vi "Execute.vi"(8 "error in (no error)":errorcluster, 11 "Node in":refnum<class "bt_Selector.lvclass">) -> (0 "error out":errorcluster, 1 "Status":T1, 3 "Node out":refnum<class "bt_Selector.lvclass">)   [LabVIEW 2021, in "BT.lvlib" / "bt_Selector.lvclass"]
uses:
  bt_Selector.lvclass
  bt_Selector.lvclass/bt_Selector.ctl
  abs_Node/Status.ctl
  abs_Node/bt_Node.lvclass
  abs_Composite/bt_Composite.lvclass
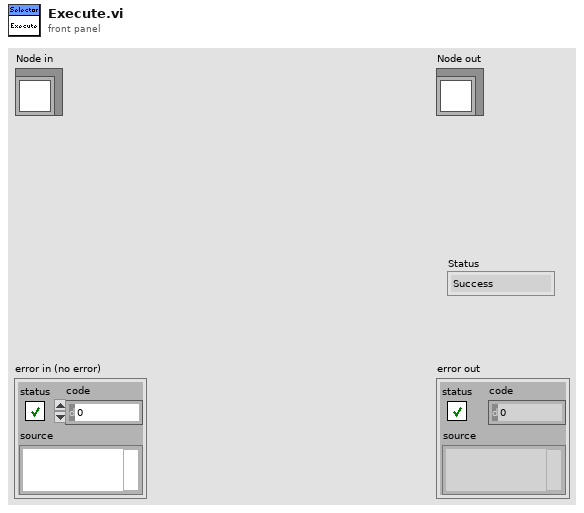
[diagram p1: front panel]
types:
  T1 = typedef "BT.lvlib/bt_Node.lvclass/Status.ctl" = enum16{"Success", "Failure", "Running"}
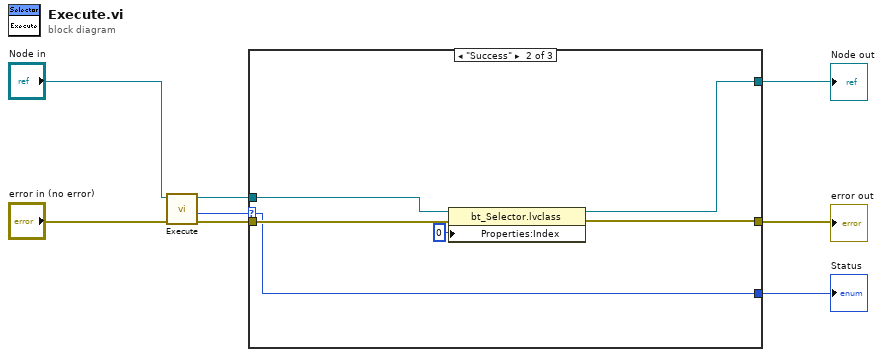
[diagram p0: block diagram]
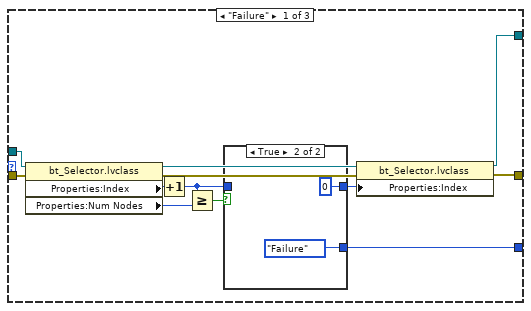
[diagram p2: hidden frame]
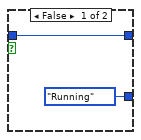
[diagram p3: hidden frame]
diagram:
  n1 = call-parent "Execute.vi"("error in (no error)"="error in (no error)", "Node in"="Node in") -> ("error out"=w3:errorcluster, "Status"=w1:T1, "Node out"=w2:refnum<class "bt_Selector.lvclass">)  [unwired: 7 in]
  n2 = case shown="\"Success\"" w1 {
    selector: w1 -> [_ w25 w31]
    tunnel: w3 -> [w18 w30 w32]
    tunnel: [w20 w29 w32] -> w5
    tunnel: w2 -> [w16 w28 w33]
    tunnel: [w19 w26 w33] -> w6
    tunnel: [w9 w25 w31] -> w4
    frame "Failure" {
      n3 = property class="bt_Selector.lvclass"(reference=w16, error in=w18) -> (reference out=w15:refnum<class "bt_Selector.lvclass">, error out=w17:errorcluster, "Properties:Index"=w14:i32, "Properties:Num Nodes"=w13:i32)
      n4 = Increment(x=w14) -> (x+1=w12:i32)
      n5 = Greater Or Equal?(x=w12, y=w13) -> (x >= y?=w10:bool)
      n6 = case shown="True" w10 {
        tunnel: w12 -> [w22 _]
        tunnel: [w22 0] -> w11
        tunnel: [Status."Running" ("Status") Status."Failure" ("Status")] -> w9
        frame False {
        }
        frame True {
        }
      }
      n7 = property class="bt_Selector.lvclass"(reference=w15, error in=w17, "Properties:Index"=w11) -> (reference out=w19:refnum<class "bt_Selector.lvclass">, error out=w20:errorcluster)
    }
    frame "Success" {
      n8 = property class="bt_Selector.lvclass"(reference=w28, error in=w30, "Properties:Index"=0 ("Index")) -> (reference out=w26:refnum<class "bt_Selector.lvclass">, error out=w29:errorcluster)
    }
    frame "Running" {
    }
  }
  "error out" <- w5
  "Node out" <- w6
  "Status" <- w4
